vi "W3Q1.vi"() -> ()   [LabVIEW 2023]
panel:
  out "Boolean 4":bool
  out "Boolean 3":bool
  out "Boolean 2":bool
  out "Boolean":bool
  in  "Color Box":u32(colorbox)
  out "Text Indicator":string
  in  "Knob":dbl(knob) scale=0.0..10.0
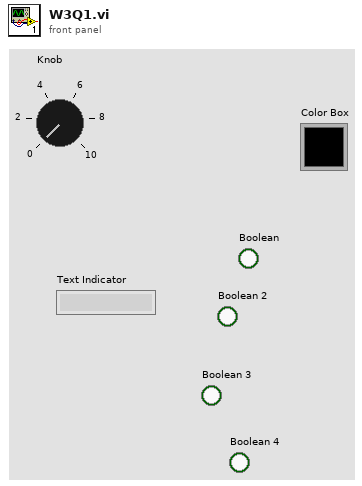
[diagram p1: front panel]
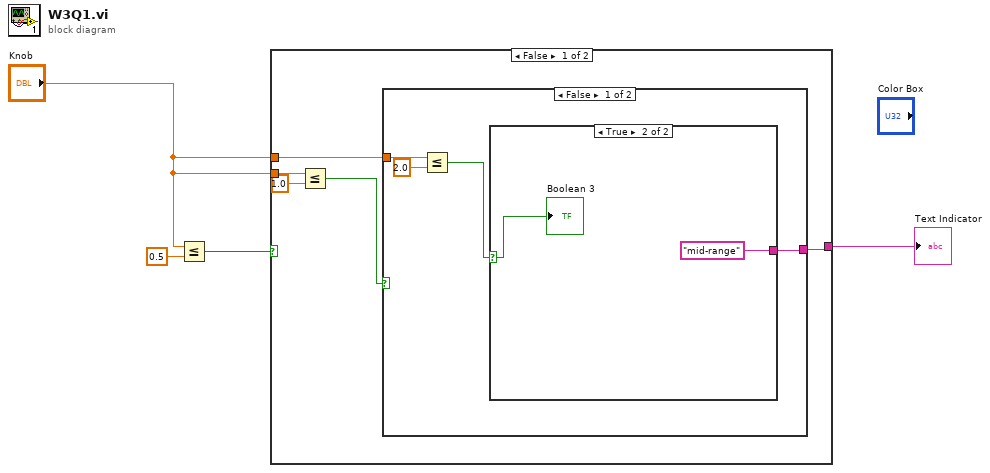
[diagram p0: block diagram]
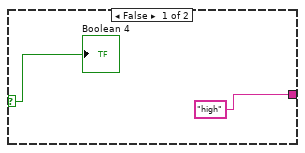
[diagram p2: hidden frame]
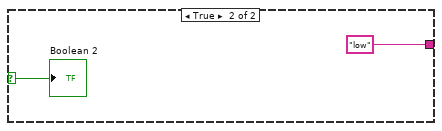
[diagram p3: hidden frame]
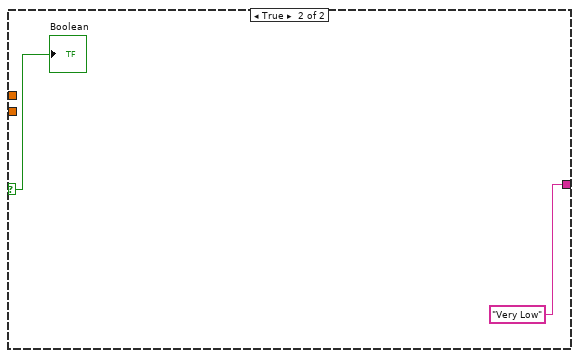
[diagram p4: hidden frame]
diagram:
  n1 = Less Or Equal?(x="Knob", y=0.5) -> (x <= y?=w2:bool)
  n2 = case shown="False" w2 {
    selector: w2 -> [_ w20]
    tunnel: [w5 "Very Low"] -> w4
    tunnel: "Knob" -> [w8 _]
    tunnel: "Knob" -> [w6 _]
    frame False {
      n3 = Less Or Equal?(x=w8, y=1.0) -> (x <= y?=w9:bool)
      n4 = case shown="False" w9 {
        selector: w9 -> [_ w18]
        tunnel: [w10 "low"] -> w5
        tunnel: w6 -> [w13 _]
        frame False {
          n5 = Less Or Equal?(x=w13, y=2.0) -> (x <= y?=w11:bool)
          n6 = case shown="True" w11 {
            selector: w11 -> [w15 w17]
            tunnel: ["high" "mid-range"] -> w10
            frame False {
              "Boolean 4" <- w15
            }
            frame True {
              "Boolean 3" <- w17
            }
          }
        }
        frame True {
          "Boolean 2" <- w18
        }
      }
    }
    frame True {
      "Boolean" <- w20
    }
  }
  "Text Indicator" <- w4
